vi "CRYImp wiz global.vi"() -> ()   [LabVIEW 2013]
panel:
  in  "std header":string[][](array[string])
  in  "header names":string[](array[string])
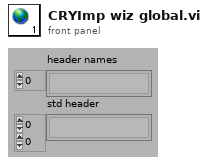
[diagram p1: front panel]
diagram:
